vi "FdxCmdTxQueueCreateCvi.vi"(8 "error in":errorcluster, 9 "QueueSizeIn":u32, 11 "InstrumentHandle_port":u32) -> (0 "error out":errorcluster, 1 "TxQueueInfo":cluster{"QueueBaseAddr":u32, "QueueSizeOut":u32}, 3 "InstrumentHandle_port":u32)   [LabVIEW 2020, in "AIM664LV.lvlib"]
doc: "This function is used to create a queue of AFDX Frames. This Queue is the input for the Generic or Replay Transmit Mode. Only one Transmit Queue can be created for one port."
uses:
  AIM664LV.lvlib
  AFDX_LibraryAdmin/FdxGlobalDllPath.vi
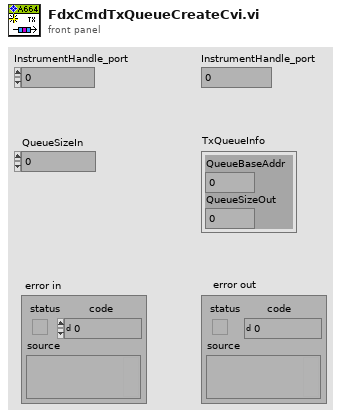
[diagram p1: front panel]
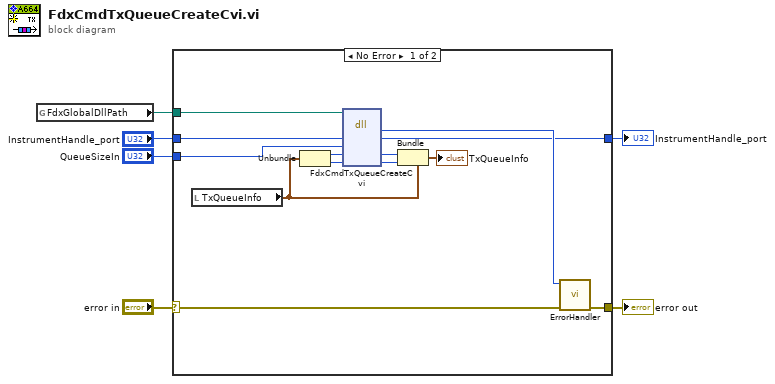
[diagram p0: block diagram]
diagram:
  n1 = global read "FdxGlobalDllPath.vi" "FdxGlobalDllPath"() -> (w4:path)
  n2 = case shown="No Error" "error in" {
    selector: "error in" -> [w18 w21]
    tunnel: [w19 w21] -> w6
    tunnel: w4 -> [w10 _]
    tunnel: "InstrumentHandle_port" -> [w9 w20]
    tunnel: [w8 w20] -> w2
    tunnel: "QueueSizeIn" -> [w7 _]
    frame No Error {
      n3 = local read "TxQueueInfo"() -> (w13:cluster{"QueueBaseAddr":u32, "QueueSizeOut":u32})
      n4 = Unbundle(w13) -> ("QueueBaseAddr"=w12:u32, "QueueSizeOut"=w11:u32)
      n5 = dll-call lib="aim_fdx.19.dll" fn="FdxCmdTxQueueCreateCvi"(path in=w10, "InstrumentHandle"=w9, "QueueSizeIn"=w7, "QueueBaseAddr"=w12, "QueueSizeOut"=w11) -> ("status"=w17:i32, "InstrumentHandle"=w8:u32, "QueueBaseAddr"=w15:u32, "QueueSizeOut"=w14:u32)  [unwired: 3 in, 2 out]
      n6 = Bundle(cluster=w13, "QueueBaseAddr"=w15, "QueueSizeOut"=w14) -> (→"TxQueueInfo":cluster{"QueueBaseAddr":u32, "QueueSizeOut":u32})
      n7 = call "ErrorHandler.vi"("error in"=w18, "AIM Error"=w17) -> ("error out"=w19:errorcluster)  [unwired: 9 in]
    }
    frame Error {
    }
  }
  "error out" <- w6
  "InstrumentHandle_port" <- w2
